vi "PTScanner.form scan tree.vi"(0 "VI Refnum":refnum<vi>, 2 "Scan Tree Ref":refnum<vi>, 5 "error in (no error)":errorcluster) -> (14 "VI Refnum out":refnum<vi>, 19 "error out":errorcluster)   [LabVIEW 2014, in "PTScanner.lvlib"]
uses:
  PTScanner.lvlib
panel:
  in  "Item":T1
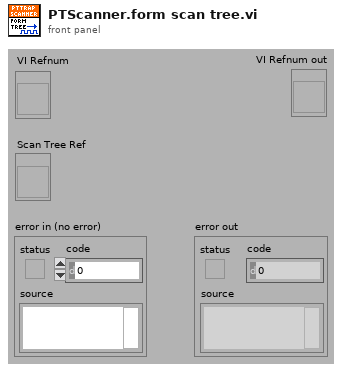
[diagram p1: front panel]
types:
  T1 = cluster{"Left Cell String":string, "Child Text":string[], "Child Tag":string, "Item Indent":i32, "Child Only?":bool, "Glyph Index":i32}
  T2 = typedef "PTScanner.lvlib/PTScanner.i attribute.ctl" = cluster{"Object cmds":T3[], "Steps":cluster{"Finished":bool, "cmd setup":T4[]}[], "curStep":i32, "DIM IDs":cluster{"AllFinished":i32, "Finished":i32, "curStep":i32, "nofSteps":i32, "NomValues":i32[], "1D-Min":i32, "1D-Max":i32, "Dimensions":i32, "MaxDimensions":i32, "ScanedDeviceNames":i32[]}, "All Finished":bool, "DIMs in use":string[], "Running":bool, "Scan Delay":u32, "loop":bool, "Paused":bool, "Formed":bool}
  T3 = typedef "PTScanner.lvlib/PTScanner.obj parameters.ctl" = cluster{"object":string, "DIM address":string, "method":string, "data descriptor":string, "method parameters":cluster{"Name":string, "Descr":string, "Value":string, "Value?":bool}[], "Call Mode":enum16{"Simple DIM", "Synchronous"}, "actValue":dbl, "Centroid":dbl, "Minus Delta":dbl, "Plus Delta":dbl, "increment":dbl, "DIM Status":cluster{"no link":bool, "quality":i32, "Time Stamp":timestamp}, "range":dbl, "DIMChannelIndex":i32}
  T4 = typedef "PTScanner.lvlib/PTScanner.step obj parameters.ctl" = cluster{"obj index":i32, "nomValue":dbl, "fulfilled":bool}
  T5 = cluster{"Left Cell String":string, "Child Text":string[], "Child Tag":string, "Item Indent":i32, "Child Only?":bool, "Glyph Index":i32}[]
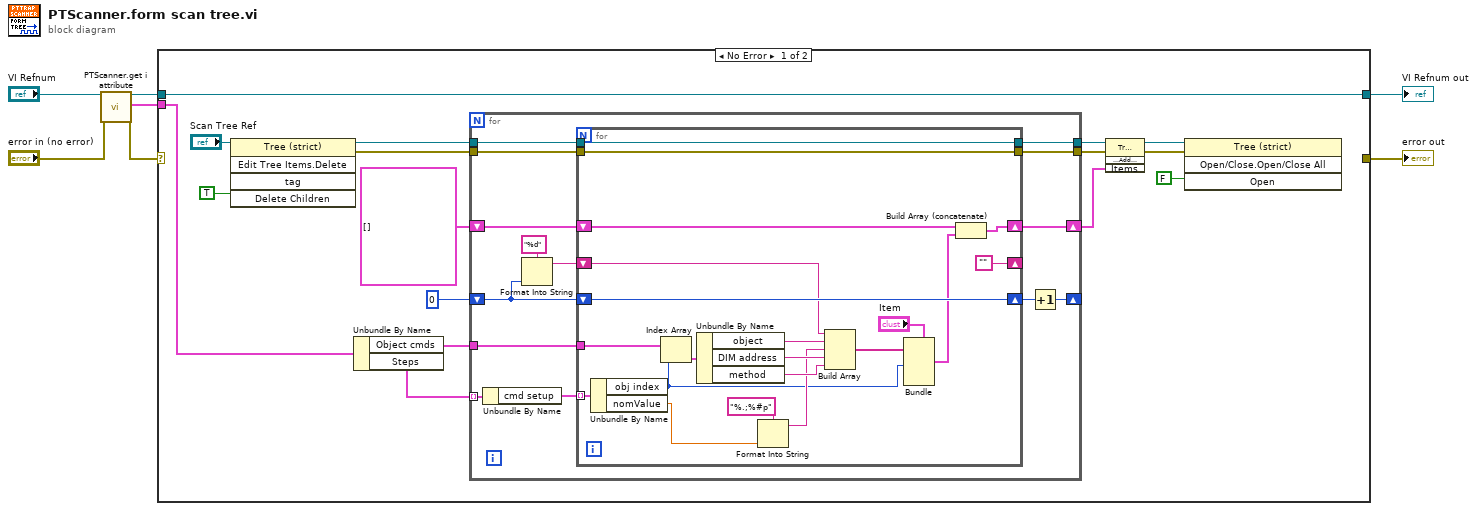
[diagram p0: block diagram]
diagram:
  n1 = call "PTScanner.get i attribute.vi"("i ref in"="VI Refnum", "error in (no error)"="error in (no error)") -> ("i ref out"=w3:refnum<vi>, "i attribute"=w5:T2, "error out"=w4:errorcluster)  [unwired: 15 in]
  n2 = case shown="No Error" w4 {
    selector: w4 -> [_ w58]
    tunnel: w5 -> [w23 _]
    tunnel: w3 -> [w20 w59]
    tunnel: [w20 w59] -> w2
    tunnel: [_ w58] -> w1
    frame No Error {
      n3 = invoke on="Invoke Node" class="Tree (strict)" method="Edit Tree Items.Delete"(reference="Scan Tree Ref", "Delete Children"=TRUE ("Delete Children?")) -> (reference out=w16:refnum<vi>, error out=w17:errorcluster)  [unwired: 3 in, 3 out]
      n4 = Unbundle By Name(w23) -> ("Object cmds"=w22:T3[], "Steps"=w21:cluster{"Finished":bool, "cmd setup":T4[]}[])
      n5 = for {
        tunnel: w21 -> [w37] mode=indexing
        tunnel: w22 -> [w35]
        tunnel: w17 -> [w34]
        tunnel: [w33] -> w13
        tunnel: w16 -> [w32]
        tunnel: [w31] -> w8
        shift-right: [w29] -> _
        shift-left: 0 -> [w26]
        shift-right: [w28] -> w11
        shift-left: T5 [] -> [w27]
        n6 = Unbundle By Name(w37) -> ("cmd setup"=w36:T4[])
        n7 = Format Into String(format string="%d", w26) -> (resulting string=w25:string)  [unwired: 2 in, 1 out]
        n8 = for {
          tunnel: w36 -> [w57] mode=indexing
          tunnel: w35 -> [w56]
          tunnel: w34 -> [w44]
          tunnel: [w44] -> w33
          tunnel: w32 -> [w45]
          tunnel: [w45] -> w31
          shift-right: [w49] -> w30
          shift-left: w26 -> [w49]
          shift-right: [w42] -> w28
          shift-left: w27 -> [w41]
          shift-right: [""] -> _
          shift-left: w25 -> [w39]
          n9 = Unbundle By Name(w57) -> ("obj index"=w46:i32, "nomValue"=w50:dbl)
          n10 = Index Array(array=w56, index=w46) -> (element=w55:T3)
          n11 = Unbundle By Name(w55) -> ("object"=w40:string, "DIM address"=w54:string, "method"=w53:string)
          n12 = Format Into String(format string="%.;%#p", w50) -> (resulting string=w51:string)  [unwired: 2 in, 1 out]
          n13 = Build Array(w39, w40, w51, w54, w53) -> (w47:string[])
          n14 = Bundle(cluster="Item", "Child Text"=w47, "Item Indent"=w46) -> (w43:T1)  [unwired: 4 in]
          n15 = Build Array (concatenate)(w41, w43) -> (w42:T5)
        }
        n16 = Increment(x=w30) -> (x+1=w29:i32)
      }
      n17 = invoke on="Invoke Node" class="Tree (strict)" method="Edit Tree Items.Add Multiple Items to End"(reference=w8, error in=w13, "Items"=w11) -> (reference out=w14:refnum<vi>, error out=w12:errorcluster)  [unwired: 1 in, 2 out]
      n18 = invoke on="Invoke Node" class="Tree (strict)" method="Open/Close.Open/Close All"(reference=w14, error in=w12, "Open"=FALSE ("Open?")) -> ()  [unwired: 1 in, 4 out]
    }
    frame Error {
    }
  }
  "error out" <- w1
  "VI Refnum out" <- w2
